vi "TriggerCheck.vi"(7 "SamplesOverThreshold (<255)":u8, 9 "TriggerLevel":i16, 11 "Acceleration":i16) -> (3 "Trigger?":bool)   [LabVIEW 2020]
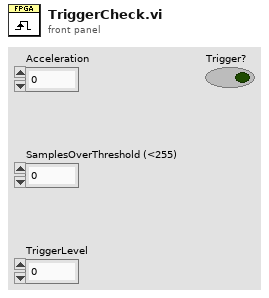
[diagram p1: front panel]
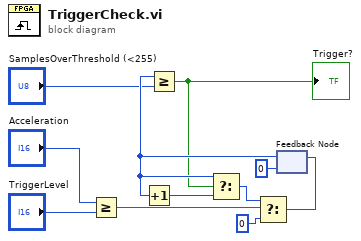
[diagram p0: block diagram]
diagram:
  n1 = Greater Or Equal?(x="Acceleration", y="TriggerLevel") -> (x >= y?=w3:bool)
  n2 = feedback #1(u8 0 ("f")) -> (w10:u8)
  n3 = Increment(x=w10) -> (x+1=w9:u8)
  n4 = Greater Or Equal?(x=w10, y="SamplesOverThreshold (<255)") -> (x >= y?=w8:bool)
  "Trigger?" <- w8
  n5 = Select(t=w10, s=w8, f=w9) -> (s? t:f=w11:u8)
  n6 = Select(t=w11, s=w3, f=u8 0) -> (s? t:f=w5:u8)
  n7 = feedback-in #1(w5) -> ()
